vi "init.vi"(8 "error in (no error)":errorcluster, 9 "Default Data":variant, 10 "Allowed Robot Modes":string[](array[string]), 11 "Name":string) -> (0 "error out":errorcluster, 3 "Command out":refnum<class "Command.lvclass">)   [LabVIEW 2017, in "Command.lvclass"]
uses:
  <userlib>/836-Library/Robot/Command/Command.lvclass
  <userlib>/836-Library/Robot/Command/Command.lvclass/Command.ctl
  <vilib>/Utility/error.llb/Error Cluster From Error Code.vi
  <vilib>/ErrorRing/Error Ring.xnode
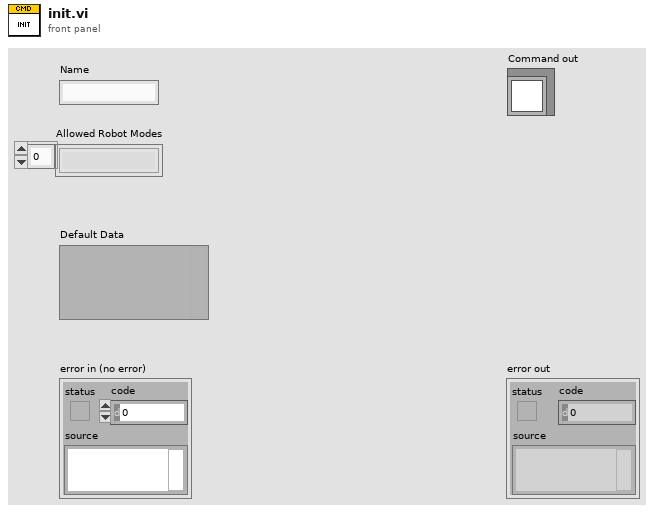
[diagram p1: front panel]
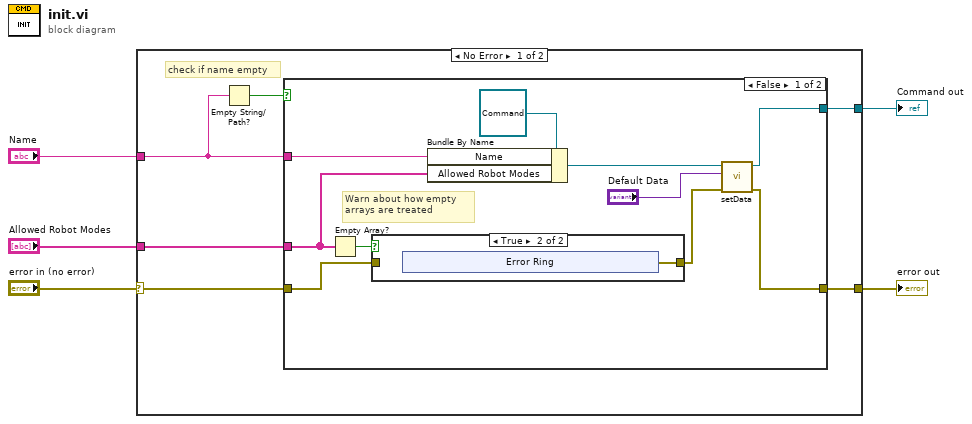
[diagram p0: block diagram]
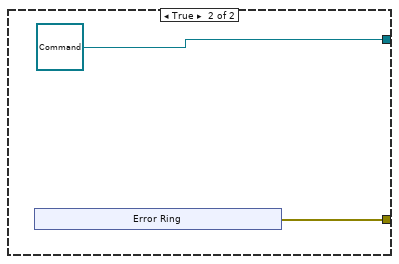
[diagram p3: hidden frame]
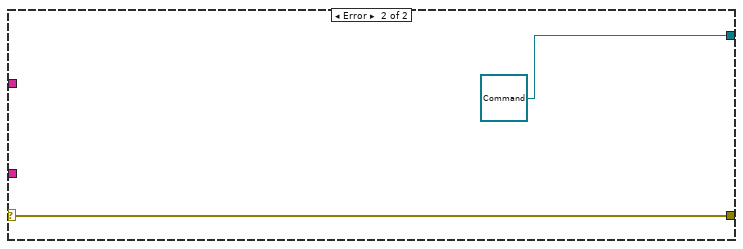
[diagram p4: hidden frame]
diagram:
  n1 = case shown="No Error" "error in (no error)" {
    selector: "error in (no error)" -> [w10 w37]
    tunnel: [w9 w37] -> w4
    tunnel: "Name" -> [w8 _]
    tunnel: "Allowed Robot Modes" -> [w7 _]
    tunnel: [w6 refnum<class "Command.lvclass"> refnum ("Command.lvclass")] -> w1
    frame No Error {
      # "check if name empty"
      n2 = Empty String/Path?(string/path=w8) -> (empty?=w11:bool)
      n3 = case shown="False" w11 {
        tunnel: w10 -> [w15 _]
        tunnel: [w12 w29] -> w9
        tunnel: w8 -> [w20 _]
        tunnel: w7 -> [w17 _]
        tunnel: [w18 refnum<class "Command.lvclass"> refnum ("Command.lvclass")] -> w6
        frame False {
          # "Warn about how empty \narrays are treated"
          n4 = Empty Array?(array=w17) -> (empty?=w16:bool)
          n5 = case shown="True" w16 {
            tunnel: w15 -> [w22 _]
            tunnel: [w22 w23] -> w14
            frame False {
            }
            frame True {
              n6 = xnode "Error Ring"() -> ("error out"=w23:errorcluster)
            }
          }
          n7 = Bundle By Name(cluster=refnum<class "Command.lvclass"> refnum ("Command.lvclass"), "Name"=w20, "Allowed Robot Modes"=w17) -> (w19:refnum<class "Command.lvclass">)
          n8 = call <userlib>:"setData.vi"("error in (no error)"=w14, "Data"="Default Data", "Command in"=w19) -> ("error out"=w12:errorcluster, "Command out"=w18:refnum<class "Command.lvclass">)  [unwired: 7 in]
        }
        frame True {
          n9 = xnode "Error Ring"() -> ("error out"=w29:errorcluster)
        }
      }
    }
    frame Error {
    }
  }
  "error out" <- w4
  "Command out" <- w1
